vi "from string.vi"(8 "error in":errorcluster, 9 "data":string, 10 "version":string, 11 "SQLite configuration in":refnum<class "SQLite configuration.lvclass">) -> (0 "error out":errorcluster, 3 "SQLite configuration out":refnum<class "SQLite configuration.lvclass">)   [LabVIEW 2014, in "SQLite configuration.lvclass"]
doc: "Provides an interface for loading a module configuration from a file or other serialized data source. It is recommended that all children of this class store data in two sets--data required for its own initialization, and any data required for parent initialization--and that each implementation uses the <b>Call Parent Method</b> primitive to de-serialize parent information. As a result, it is expected that every module configuration class calls <b>component configuration.lvclass:From String.vi</b>."
uses:
  SQLite configuration.lvclass
  <vilib>/NI/Tag Bus Module Framework/channel/TBM channel.lvclass
  Line.ctl
  SQLite configuration.lvclass/SQLite configuration.ctl
  <vilib>/NI/Tag Bus Module Framework/module configuration/TBM module configuration.lvclass
  <vilib>/NI/Configuration Framework/serializable configuration/NISE_CEF_serializable configuration.lvclass
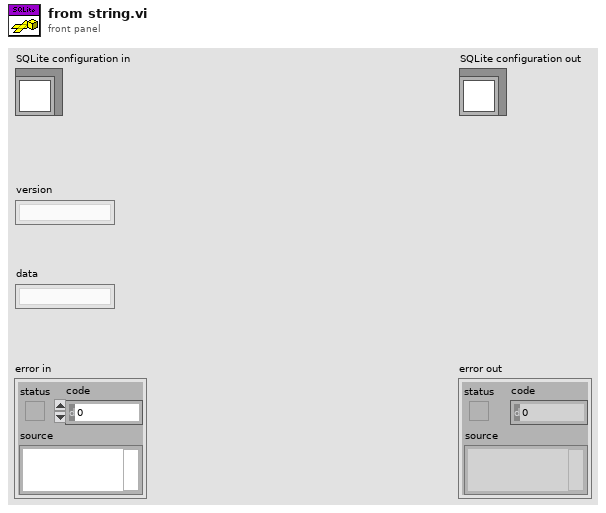
[diagram p1: front panel]
types:
  T1 = typedef "SQLite configuration.lvclass/Line.ctl" = cluster{"channel":refnum<class "TBM channel.lvclass">}
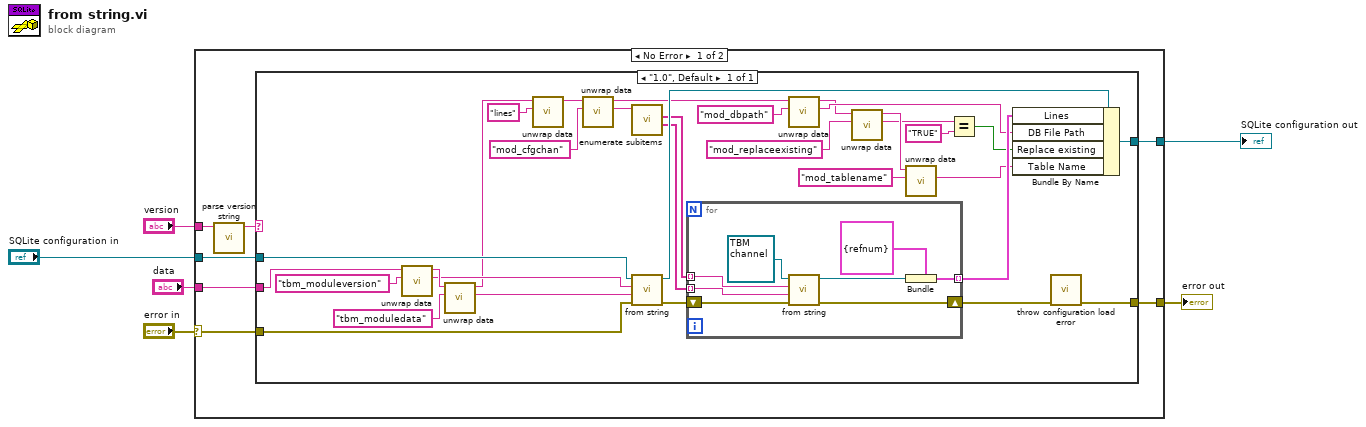
[diagram p0: block diagram]
diagram:
  n1 = case shown="No Error" "error in" {
    selector: "error in" -> [w7 w55]
    tunnel: "data" -> [w13 _]
    tunnel: "SQLite configuration in" -> [w12 w54]
    tunnel: [w11 w54] -> w5
    tunnel: [w10 w55] -> w4
    tunnel: "version" -> [w9 _]
    frame No Error {
      n2 = call <vilib>:"parse version string.vi"("full version"=w9) -> ("major.minor version"=w8:string)  [unwired: 7 in, 3 out]
      n3 = case shown="\"1.0\", Default" w8 {
        tunnel: w13 -> [w42]
        tunnel: w7 -> [w41]
        tunnel: w12 -> [w45]
        tunnel: [w33] -> w11
        tunnel: [w44] -> w10
        frame "1.0", Default {
          n4 = call <vilib>:"unwrap data.vi"("identifier"="tbm_moduleversion" ("additional identifier"), "data to unwrap"=w42) -> ("unwrapped data"=w37:string, "remaining string"=w43:string)  [unwired: 8 in]
          n5 = call <vilib>:"unwrap data.vi"("identifier"="tbm_moduledata" ("additional identifier"), "data to unwrap"=w43) -> ("unwrapped data"=w39:string, "remaining string"=w36:string)  [unwired: 8 in]
          n6 = call <vilib>:"unwrap data.vi"("identifier"="lines" ("additional identifier"), "data to unwrap"=w36) -> ("remaining string"=w32:string)  [unwired: 8 in, 1 out]
          n7 = call <vilib>:"unwrap data.vi"("identifier"="mod_cfgchan", "data to unwrap"=w32) -> ("unwrapped data"=w27:string, "remaining string"=w24:string)  [unwired: 8 in]
          n8 = call <vilib>:"enumerate subitems.vi"("data to enumerate"=w27) -> ("associated data"=w29:string[], "discovered subitems"=w30:string[])  [unwired: 8 in, 1 out]
          n9 = call-parent "from string.vi"("error in"=w41, "data"=w39, "version"=w37, "module configuration in"=w45) -> ("error out"=w28:errorcluster, "module configuration out"=w34:refnum<class "SQLite configuration.lvclass">)  [unwired: 6 in]
          n10 = for {
            shift-right: [w53] -> w25
            shift-left: w28 -> [w52]
            tunnel: w30 -> [w51] mode=indexing
            tunnel: w29 -> [w50] mode=indexing
            tunnel: [w46] -> w26 mode=indexing
            n11 = call-dynamic "from string.vi"("error in"=w52, "channel data"=w50, "identifier"=w51, "channel in"=refnum<class "TBM channel.lvclass"> refnum) -> ("error out"=w53:errorcluster, "channel out"=w47:refnum<class "TBM channel.lvclass">)  [unwired: 6 in]
            n12 = Bundle(cluster=T1 {"channel"=refnum} ("Line"), "channel"=w47) -> (w46:T1)
          }
          n13 = call <vilib>:"unwrap data.vi"("identifier"="mod_dbpath", "data to unwrap"=w24) -> ("unwrapped data"=w22:string, "remaining string"=w21:string)  [unwired: 8 in]
          n14 = call <vilib>:"unwrap data.vi"("identifier"="mod_replaceexisting", "data to unwrap"=w21) -> ("unwrapped data"=w16:string, "remaining string"=w19:string)  [unwired: 8 in]
          n15 = call <vilib>:"unwrap data.vi"("identifier"="mod_tablename", "data to unwrap"=w19) -> ("unwrapped data"=w17:string)  [unwired: 8 in, 1 out]
          n16 = Equal?(x=w16, y="TRUE") -> (x = y?=w14:bool)
          n17 = Bundle By Name(cluster=w34, "Lines"=w26, "DB File Path"=w22, "Replace existing"=w14, "Table Name"=w17) -> (w33:refnum<class "SQLite configuration.lvclass">)
          n18 = call <vilib>:"throw configuration load error.vi"("error in"=w25) -> ("error out"=w44:errorcluster)  [unwired: 10 in]
        }
      }
    }
    frame Error {
    }
  }
  "error out" <- w4
  "SQLite configuration out" <- w5
